vi "Listbox FGV - Serial Bus.vi"(0 "MulticolumnListbox in":refnum<vi>, 2 "Enum":enum16{"Init", "Replace", "Clear", "Release"}(ring), 7 "Array":string[](array[string])=["0", "0", "0"], 11 "error in":errorcluster) -> (6 "Index":i32, 15 "error out":errorcluster)   [LabVIEW 2011]
uses:
  <vilib>/Utility/miscctls.llb/LVRowAndColumnUnsignedTypeDef.ctl
  <vilib>/Utility/miscctls.llb/LVRowAndColumnTypeDef.ctl
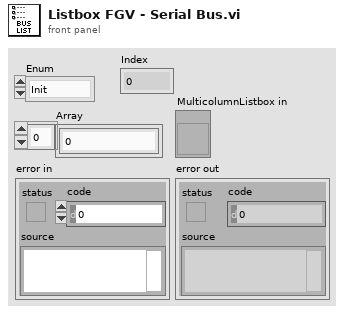
[diagram p1: front panel]
types:
  T1 = typedef "LVRowAndColumnTypeDef.ctl" = cluster{"Row":i32, "Column":i32}
  T2 = typedef "LVRowAndColumnUnsignedTypeDef.ctl" = cluster{"Row":u32, "Column":u32}
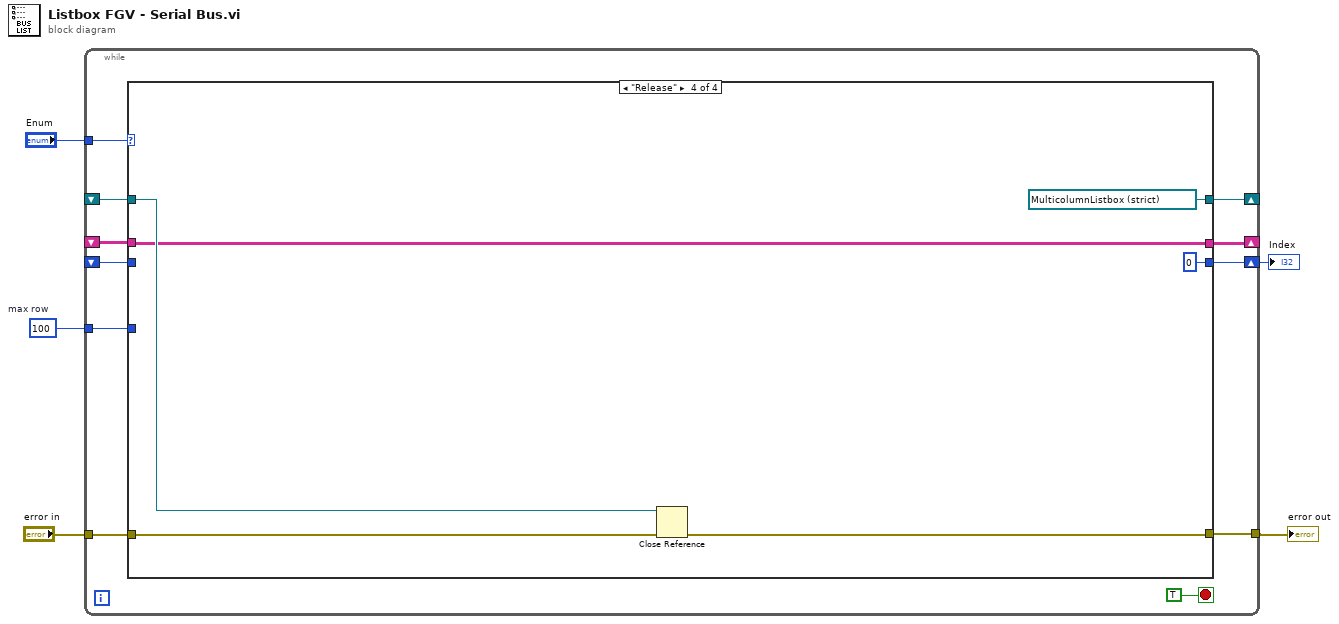
[diagram p0: block diagram]
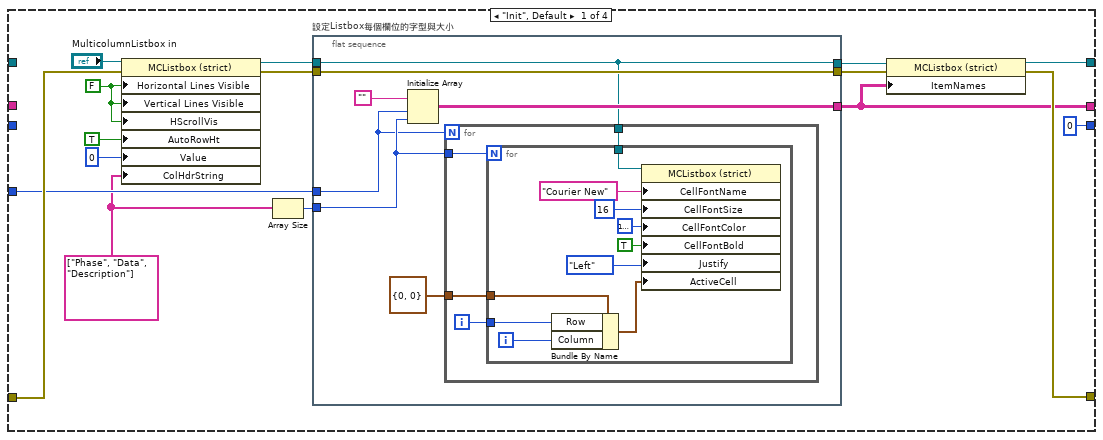
[diagram p2: hidden frame]
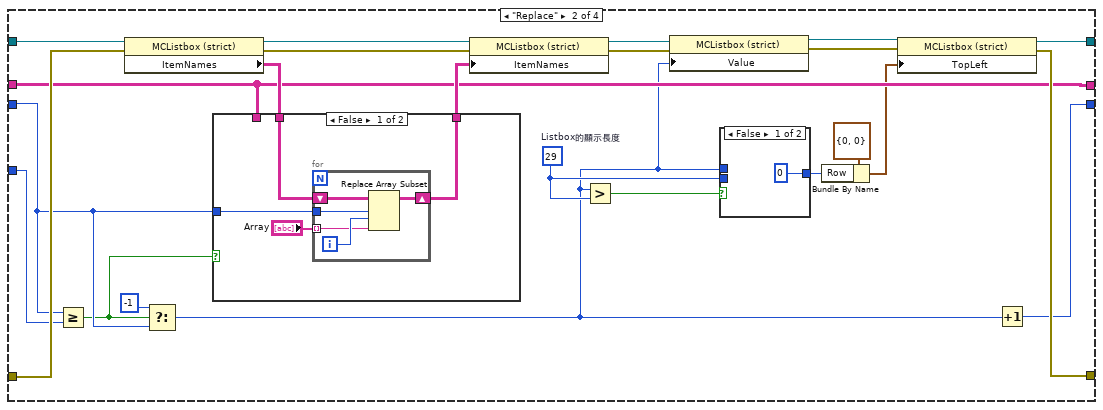
[diagram p3: hidden frame]
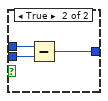
[diagram p4: hidden frame]
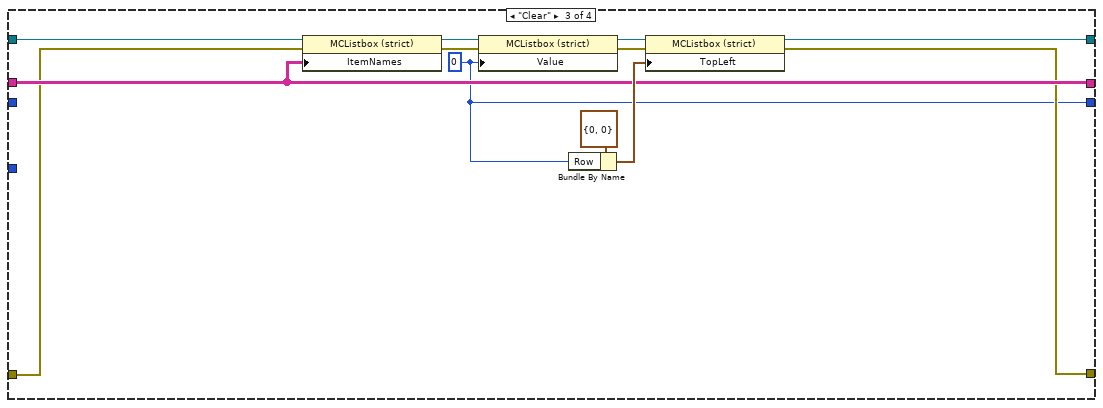
[diagram p6: hidden frame]
diagram:
  w2 = 100  # max row
  n1 = while {
    shift-right: [w15] -> _
    shift-left: _ -> [w14]
    tunnel: "Enum" -> [w13]
    tunnel: "error in" -> [w12]
    tunnel: [w11] -> w3
    shift-right: [w10] -> _
    shift-left: _ -> [w9]
    shift-right: [w7] -> w1
    shift-left: _ -> [w8]
    tunnel: w2 -> [w6]
    stop <- TRUE stop-if-true
    n2 = case shown="\"Release\"" w13 {
      tunnel: w14 -> [_ w76 w96 w107]
      tunnel: [w28 w70 w97 refnum<vi> refnum ("MulticolumnListbox in")] -> w15
      tunnel: w12 -> [w25 w75 w94 w109]
      tunnel: [w24 w69 w93 w108] -> w11
      tunnel: [w23 w65 w95 w104] -> w10
      tunnel: w9 -> [_ w65 w95 w104]
      tunnel: w8 -> [_ w67 _ _]
      tunnel: [0 w59 w92 0 ("Value")] -> w7
      tunnel: w6 -> [w20 w64 _ _]
      frame "Init", Default {
        w21 = FALSE
        w18 = string[] ["Phase", "Data", "Description"] ("Column Headers")
        n3 = property on="Property Node" class="MCListbox (strict)"(reference="MulticolumnListbox in", error in=w25, "Horizontal Lines Visible"=w21, "Vertical Lines Visible"=w21, "HScrollVis"=w21, "AutoRowHt"=TRUE ("Autosizing Row Height"), "Value"=0, "ColHdrString"=w18) -> (reference out=w31:refnum<vi>, error out=w29:errorcluster)
        n4 = Array Size(array=w18) -> (size(s)=w27:i32)
        n5 = flat-sequence "設定Listbox每個欄位的字型與大小" {
          tunnel: w29 -> [w37]
          tunnel: [w37] -> w30
          tunnel: [w36] -> w23
          tunnel: w31 -> [w35]
          tunnel: [w35] -> w32
          tunnel: w27 -> [w34]
          tunnel: w20 -> [w33]
          frame #0 {
            n6 = Initialize Array("", w33, w34) -> (w36:string[][])
            n7 = for {
              N: w33 -> [_]
              tunnel: T1 {"Row"=0, "Column"=0} ("Active Cell:Active Cell") -> [w43]
              tunnel: w34 -> [w42]
              tunnel: w35 -> [w40]
              i -> [w41]
              n8 = for {
                N: w42 -> [_]
                tunnel: w43 -> [w51]
                tunnel: w41 -> [w50]
                tunnel: w40 -> [w49]
                i -> [w45]
                n9 = Bundle By Name(cluster=w51, "Row"=w50, "Column"=w45) -> (w46:T1)
                n10 = property on="Property Node" class="MCListbox (strict)"(reference=w49, "CellFontName"="Courier New" ("Text.Font:Name"), "CellFontSize"=u32 16 ("Text.Font:Size"), "CellFontColor"=u32 16777225, "CellFontBold"=TRUE ("Active Cell:Cell Font:Bold"), "Justify"=enum16{"Left", "Center", "Right"}."Left" ("Active Cell:Cell Justification"), "ActiveCell"=w46) -> ()  [unwired: 1 in, 2 out]
              }
            }
          }
        }
        n11 = property on="Property Node" class="MCListbox (strict)"(reference=w32, error in=w30, "ItemNames"=w23) -> (reference out=w28:refnum<vi>, error out=w24:errorcluster)
      }
      frame "Replace" {
        w62 = 29  # Listbox的顯示長度
        n12 = Greater Or Equal?(x=w67, y=w64) -> (x >= y?=w66:bool)
        n13 = property on="Property Node" class="MCListbox (strict)"(reference=w76, error in=w75) -> (reference out=w77:refnum<vi>, error out=w74:errorcluster, "ItemNames"=w73:string[][])
        n14 = Select(t=-1, s=w66, f=w67) -> (s? t:f=w56:i32)
        n15 = case shown="False" w66 {
          tunnel: w73 -> [w85 _]
          tunnel: [w83 w91] -> w72
          tunnel: w67 -> [w82 _]
          tunnel: w65 -> [_ w91]
          frame False {
            n16 = for {
              tunnel: w82 -> [w90]
              tunnel: "Array" -> [w88] mode=indexing
              shift-right: [w86] -> w83
              shift-left: w85 -> [w87]
              i -> [w89]
              n17 = Replace Array Subset(array=w87, new element=w88, index (row)=w90, index (col)=w89) -> (w86:string[][])
            }
          }
          frame True {
          }
        }
        n18 = property on="Property Node" class="MCListbox (strict)"(reference=w77, error in=w74, "ItemNames"=w72) -> (reference out=w58:refnum<vi>, error out=w57:errorcluster)
        n19 = Greater?(x=w56, y=w62) -> (0:w63:bool)
        n20 = property class="MCListbox (strict)"(reference=w58, error in=w57, "Value"=w56) -> (reference out=w54:refnum<vi>, error out=w55:errorcluster)
        n21 = case shown="False" w63 {
          tunnel: [0 ("f") w79] -> w60
          tunnel: w56 -> [_ w81]
          tunnel: w62 -> [_ w80]
          frame False {
          }
          frame True {
            n22 = Subtract(x=w81, y=w80) -> (x-y=w79:i32)
          }
        }
        n23 = Bundle By Name(cluster=T2 {"Row"=0, "Column"=0} ("Top Left Visible Cell"), "Row"=w60) -> (w61:T2)
        n24 = property class="MCListbox (strict)"(reference=w54, error in=w55, "TopLeft"=w61) -> (reference out=w70:refnum<vi>, error out=w69:errorcluster)
        n25 = Increment(x=w56) -> (x+1=w59:i32)
      }
      frame "Clear" {
        w92 = 0 ("Value")
        n26 = property on="Property Node" class="MCListbox (strict)"(reference=w96, error in=w94, "ItemNames"=w95) -> (reference out=w101:refnum<vi>, error out=w100:errorcluster)
        n27 = property class="MCListbox (strict)"(reference=w101, error in=w100, "Value"=w92) -> (reference out=w99:refnum<vi>, error out=w98:errorcluster)
        n28 = Bundle By Name(cluster=T2 {"Row"=0, "Column"=0} ("Top Left Visible Cell"), "Row"=w92) -> (w102:T2)
        n29 = property class="MCListbox (strict)"(reference=w99, error in=w98, "TopLeft"=w102) -> (reference out=w97:refnum<vi>, error out=w93:errorcluster)
      }
      frame "Release" {
        n30 = Close Reference(reference=w107, error in (no error)=w109) -> (error out=w108:errorcluster)
      }
    }
  }
  "error out" <- w3
  "Index" <- w1
